vi "CalKnee.vi"(0 "transposed array":dbl[][](array[numeric])=[[1.0, 6.1583, 18.199999999999996, 279.4207352341019], [2.0, 7.0202, 48.69999999999998, 279.0471941984746], [5.0, 9.0886, 140.86666666666667, 278.3000100182607], [10.0, 11.6588, 282.0999999999999, 278.3000100182607], [15.0, 13.571, 417.76666666666665, 277.9263668963827], [20.0, 15.136, 545.7666666666667, 277.9263668963827], [25.0, 16.537, 669.4333333333333, 278.3000100182607], [30.0, 17.834, 790.1, 278.3000100182607], [35.0, 19.055, 907.7666666666668, 278.3000100182607], [40.0, 20.223, 1022.1, 278.3000100182607], [45.0, 21.344, 1133.1, 278.3000100182607], [50.0, 22.437, 1242.1, 278.3000100182607]]) -> (1 "Knee Current":dbl, 3 "Knee Voltage":dbl)   [LabVIEW 2012]
uses:
  <vilib>/Analysis/6fits.llb/Curve Fitting Criteria.ctl
  <vilib>/Analysis/NI_AALPro.lvlib
  <vilib>/gmath/NI_Gmath.lvlib
panel:
  out "Best Linear Fit":dbl[](array[numeric])
  out "XY Graph":cluster{"all rows":dbl[], "all rows":dbl[]}(graph)
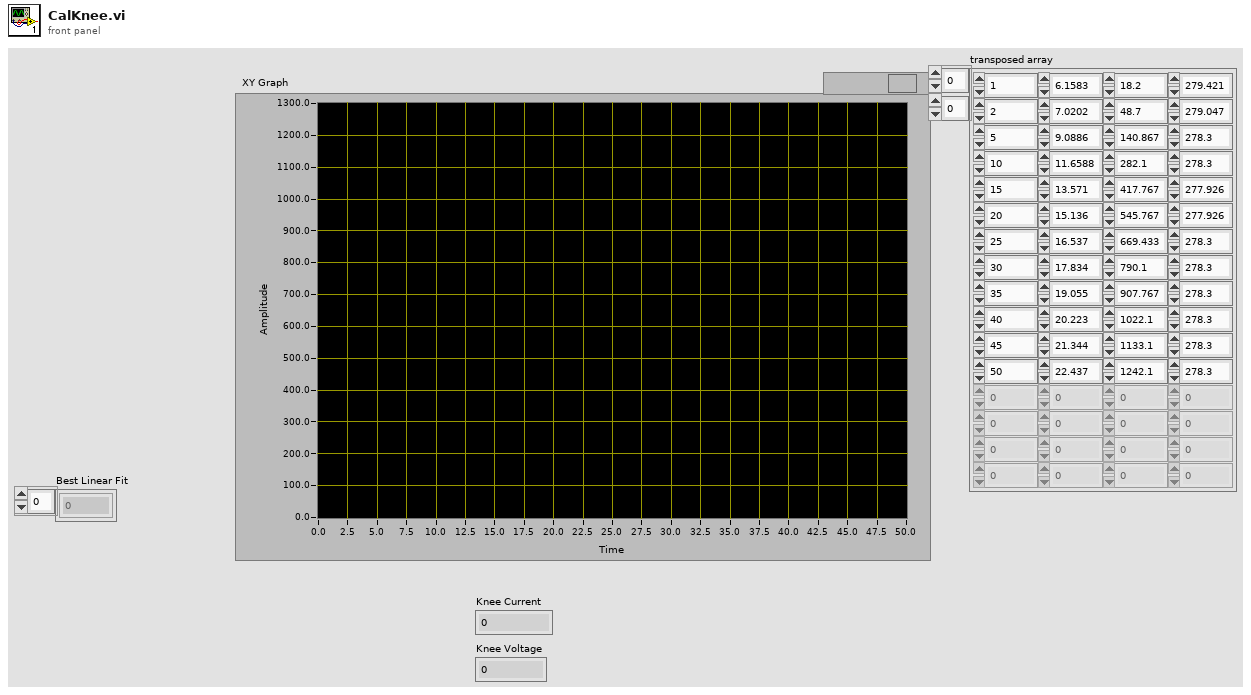
[diagram p1: front panel]
types:
  T1 = typedef "NI_AALPro.lvlib/Curve Fitting Criteria.ctl" = u16
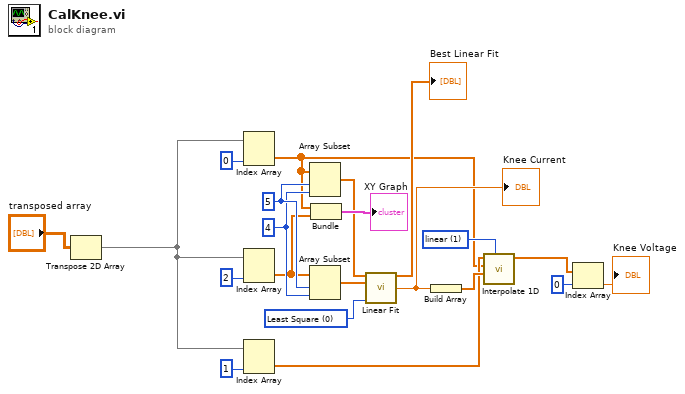
[diagram p0: block diagram]
diagram:
  w11 = 1 items=["nearest", "linear", "spline", "cubic Hermite", "Lagrange"] ("method")
  w15 = 4 ("index")
  w16 = 5 ("index")
  w18 = T1 0 items=["Least Square", "Least Absolute Residual", "Bisquare"] ("method")
  n1 = Transpose 2D Array(2D array="transposed array") -> (transposed array=w1:dbl[][])
  n2 = Index Array(array=w1, index (col)=0 ("disabled index (col)")) -> (element=w4:dbl[])  [unwired: 1 in]
  n3 = Index Array(array=w1, index (col)=2) -> (element=w3:dbl[])  [unwired: 1 in]
  n4 = Index Array(array=w1, index (col)=1 ("disabled index (col)")) -> (element=w10:dbl[])  [unwired: 1 in]
  n5 = Array Subset(array=w4, index=w16, length=w15) -> (w5:dbl[])
  n6 = Array Subset(array=w3, index=w16, length=w15) -> (w6:dbl[])
  n7 = Bundle(w4, w3) -> (→"XY Graph":cluster{dbl[], dbl[]})  [unwired: 1 in]
  n8 = call <vilib>:"Linear Fit.vi"("Y"=w5, "X"=w6, "method"=w18) -> ("Best Linear Fit"=→"Best Linear Fit":dbl[], "intercept"=w13:dbl)  [unwired: 8 in, 3 out]
  "Knee Current" <- w13
  n9 = Build Array(w13) -> (w12:dbl[])
  n10 = call <vilib>:"Interpolate 1D.vi"("method"=w11, "xi"=w12, "X"=w4, "Y"=w10) -> ("yi"=w9:dbl[])  [unwired: 5 in, 2 out]
  n11 = Index Array(array=w9, index=0) -> (element=→"Knee Voltage":dbl)
